vi "MLP Classifier.vi"(8 "error in":errorcluster) -> (0 "error out":errorcluster)   [LabVIEW 2020]
uses:
  <vilib>/Math Plots/3D Math Plots/3D Scatter/3D Scatter XCtrl/3D Scatter.xctl
  Controls/State_MLPClassifier.ctl
  Controls/Local_MLPClassifier.ctl
  Model/Supervised/MultiLayerPerceptron/MLPClassifier/MLPClassifier.lvclass
  C:/Users/cipop/TDF Dropbox/2_Technologies de France/1 - Services et Etudes/PLAIY/2 - DEV/PLAIYLAB/code/Model/Model.lvclass
  C:/Users/cipop/TDF Dropbox/2_Technologies de France/1 - Services et Etudes/PLAIY/2 - DEV/PLAIYLAB/code/Model/Supervised/MultiLayerPerceptron/MultiLayerPerceptron.lvclass
  <vilib>/Math Plots/3D Math Plots/3D Plot/3D Plot Datatype/3D Plot Datatype.lvclass
  PLAIYDISPLAY/Display/Classification/2D/Trained/Controls/2DParameters.ctl
  PLAIYDISPLAY/Display/_Controls/Datas.ctl
  PLAIYDISPLAY/Display/_Controls/PointPropertyMultipleLabel.ctl
  PLAIYDISPLAY/Display/_Controls/Style.ctl
  PLAIYDISPLAY/Display/Classification/3D/_Controls/3DParameters.ctl
  PLAIYDISPLAY/Display/Classification/2D/Predicted/Controls/PredictedParameter.ctl
  88ea5a45-d7b9-4f26-bf7b-97830e46f254.vi
  <vilib>/Utility/file.llb/Application Directory.vi
  <vilib>/Platform/system.llb/System Exec.vi
panel:
  in  "Stop":bool
  in  "TabChoice":enum32{"BTN_Train", "BTN_Predict"}(radio)
  out "Tab Control":enum32{"TRAIN", "PREDICT"}(tab)
  in  "Display_Split":enum16{"All", "Train", "Test"}(ring)
  in  "Representation":u32(ring) items=["2D", "3D"]
  out "GraphTab":enum32{"2D", "3D"}(tab)
  in  "2D":cluster{"X":i32, "Y":i32} {"Y" items=["sepal length (cm)", "sepal width (cm)", "petal length (cm)", "petal width (cm)", "Setosa/Versicolore/Virginica"]; "X" items=["sepal length (cm)", "sepal width (cm)", "petal length (cm)", "petal width (cm)", "Setosa/Versicolore/Virginica"]}
  out "Plot":cluster{"X":dbl[], "Y":dbl[]}[](graph)
  out "CursorTrain":cluster{"Y":dbl, "X":dbl}
  out "3D Scatter":refnum<class "3D Plot Datatype.lvclass">[](xcontrol) caption="Nuage 3D"
  in  "3D":cluster{"X":i32, "Y":i32, "Z":i32} {"Z" items=["sepal length (cm)", "sepal width (cm)", "petal length (cm)", "petal width (cm)", "Setosa/Versicolore/Virginica"]; "Y" items=["sepal length (cm)", "sepal width (cm)", "petal length (cm)", "petal width (cm)", "Setosa/Versicolore/Virginica"]; "X" items=["sepal length (cm)", "sepal width (cm)", "petal length (cm)", "petal width (cm)", "Setosa/Versicolore/Virginica"]}
  in  "%SplitTrain":i32(slide)=50 scale=0.0..100.0 scale format="%#_g %"
  in  "BTN_Train":bool
  in  "BTN_Sauvegarder_M":bool
  in  "BTN_Configurations":bool
  out "Good":i32 caption="Good Prediction"
  out "Bad":i32 caption="Bad Prediction"
  out "Score":dbl caption="Model Score"
  in  "BTN_Predict":bool
  in  "BTN_Load_Model":bool
  in  "PredDisplay":u32(ring) items=["Data", "Graph"]
  out "PredictTab":enum32{"Data", "Graph"}(tab)
  out "Data":dbl[][](array[numeric])
  out "Prediction":dbl[][](array[numeric])
  out "Label":string[](array[string])
  out "GraphPred":cluster{"X":dbl[], "Y":dbl[]}[](graph)
  in  "2D Pred":cluster{"X":i32, "Y":i32}={"X"=0, "Y"=1} {"Y" items=["sepal length (cm)", "sepal width (cm)", "petal length (cm)", "petal width (cm)", "Setosa/Versicolore/Virginica"]; "X" items=["sepal length (cm)", "sepal width (cm)", "petal length (cm)", "petal width (cm)", "Setosa/Versicolore/Virginica"]}
  out "CursorPred":cluster{"Y":dbl, "X":dbl}
  # "MLP Classifier Model - Training"
  # "MLP Classifier Model - Predicting"
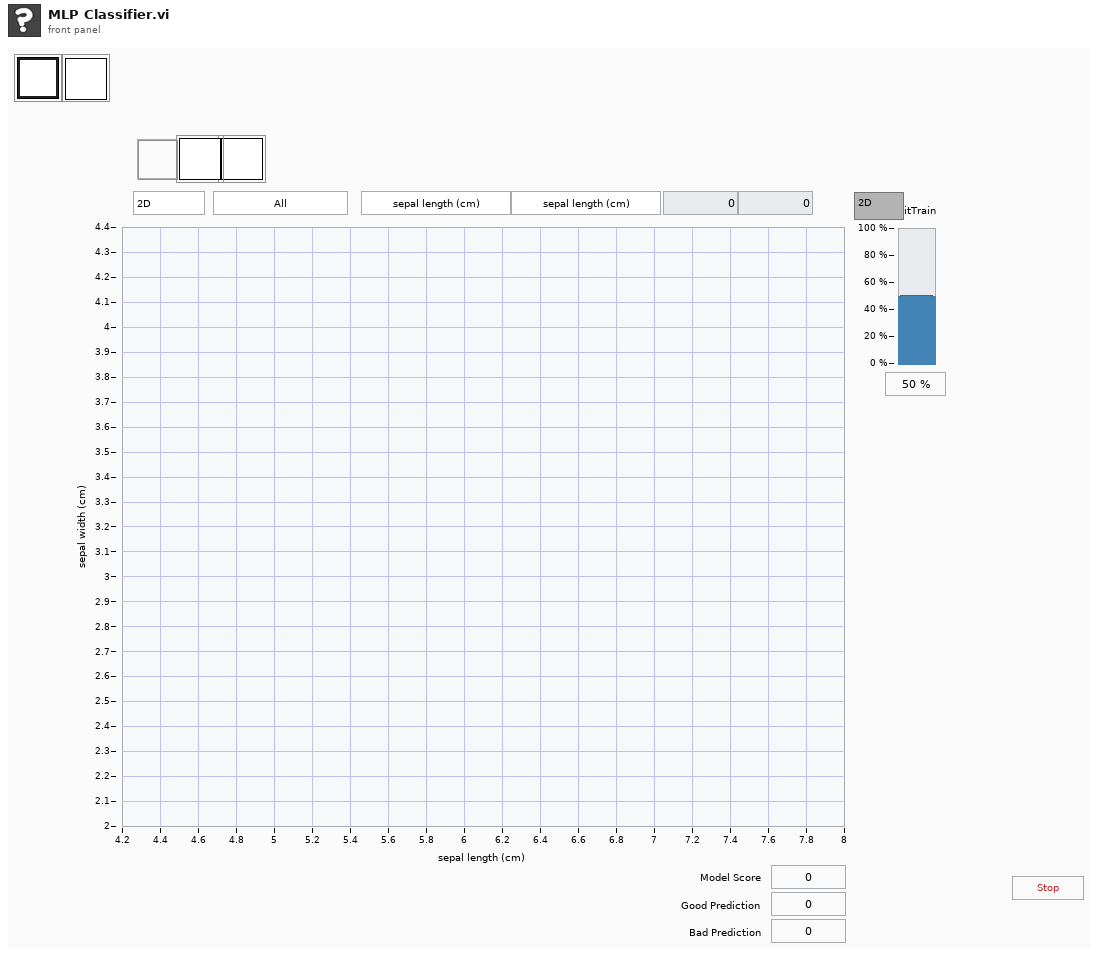
[diagram p1: front panel]
types:
  T1 = typedef "Local_MLPClassifier.ctl" = cluster{"Objet":cluster{"MLPClassifier":refnum<class "MLPClassifier.lvclass">, "3D Plot":refnum<class "3D Plot Datatype.lvclass">[]}, "Référence":cluster{"CursorTrain":refnum<vi>, "GraphPred":refnum<vi>, "GraphTrain":refnum<vi>, "Scale 2D Pred":refnum<vi>, "Scale 3D":refnum<vi>, "Scale 2D":refnum<vi>, "3D Scatter":refnum<vi>, "Data":refnum<vi>, "Prediction":refnum<vi>, "CursorPred":refnum<vi>, "Label":refnum<vi>}, "Variables":cluster{"Mode":enum32{"TRAIN", "PREDICT"}, "Model Name":string, "State":T2, "%SplitTrain":i32, "Representation":u32, "Display_Split":enum16{"All", "Train", "Test"}, "X":dbl[][], "y":dbl[][], "Split":cluster{"X Train":dbl[][], "X Test":dbl[][], "Y Train":dbl[][], "Y Test":dbl[][]}, "FitPredict":dbl[][], "Predict":dbl[][], "ScaleName":string[], "Train ? ":bool}}
  T2 = typedef "State_MLPClassifier.ctl" = enum16{"1 - Idle", "2 - Initialize", "3 - InitializeState", "4 - LoadData", "5 - ScaleName", "6 - SplitTrain", "7 - DisplayDataTrain", "8 - RefreshScale", "9 - Fit", "10 - Predict", "11 - SetParameters", "12 - SaveModel", "13 - LoadModel", "14 - DisplayDataPredict", "Error", "Exit"}
  T3 = typedef "2DParameters.ctl" = cluster{"Plot":refnum<vi>, "Data":T4, "Display":cluster{"Choice":enum16{"All", "Train", "Test"}, "Indexe":cluster{"X":i32, "Y":i32}}, "Property":T5}
  T4 = typedef "Datas.ctl" = cluster{"Split":cluster{"X Train":dbl[][], "X Test":dbl[][], "Y Train":dbl[][], "Y Test":dbl[][]}, "Predict":dbl[][]}
  T5 = typedef "PointPropertyMultipleLabel.ctl" = cluster{"Train Style":T6, "Test OK Style":T6, "Label Color":u32[], "Test NO OK":cluster{"Style":T6, "Color":u32}}
  T6 = typedef "Style.ctl" = enum16{"Empty circle", "Full circle", "Empty square", "Full square", "Cross"}
  T7 = typedef "3DParameters.ctl" = cluster{"3D Plot":refnum<class "3D Plot Datatype.lvclass">[], "3D Scatter":refnum<vi>, "Data":T4, "Display":cluster{"Choice":enum16{"All", "Train", "Test"}, "Indexe":cluster{"X":i32, "Y":i32, "Z":i32}}, "Point Property":T5, "3D Plot Datatype.lvclass":refnum<class "3D Plot Datatype.lvclass">}
  T8 = typedef "PredictedParameter.ctl" = cluster{"Plot":refnum<vi>, "Data":cluster{"X":dbl[][], "Predict":dbl[][]}, "Indexe":cluster{"X":i32, "Y":i32}, "Point Property":cluster{"Style":T6, "Label Color":u32[]}}
  T9 = cluster{"X Train":dbl[][], "X Test":dbl[][], "Y Train":dbl[][], "Y Test":dbl[][]}
  T10 = typedef "mlp_classifier_params.ctl" = cluster{"hidden_layer_sizes":dbl[], "activation":string, "solver":string, "alpha":dbl, "batch_size":cluster{"batch_size_type":string, "batch_size_int":dbl}, "learning_rate":string, "learning_rate_init":dbl, "power_t":dbl, "max_iter":dbl, "shuffle":bool, "random_state":dbl, "tol":dbl, "verbose":bool, "warm_start":bool, "momentum":dbl, "nesterovs_momentum":bool, "early_stopping":bool, "validation_fraction":dbl, "beta_1":dbl, "beta_2":dbl, "epsilon":dbl, "n_iter_no_change":dbl, "max_fun":dbl}
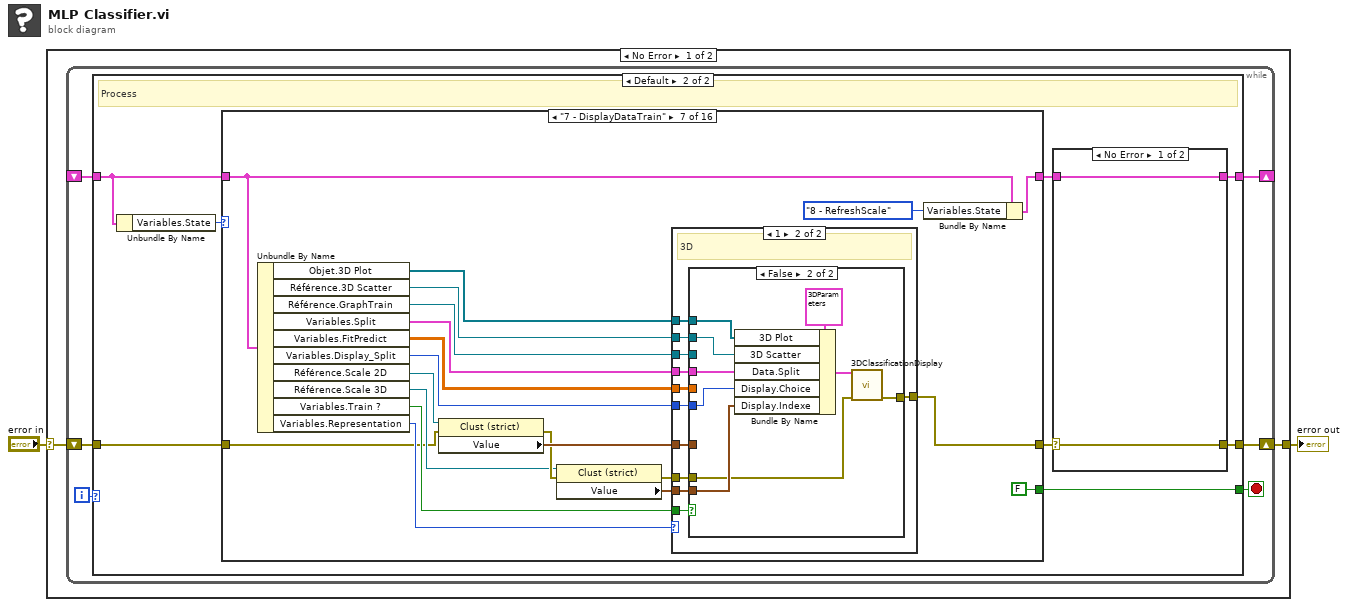
[diagram p0: block diagram]
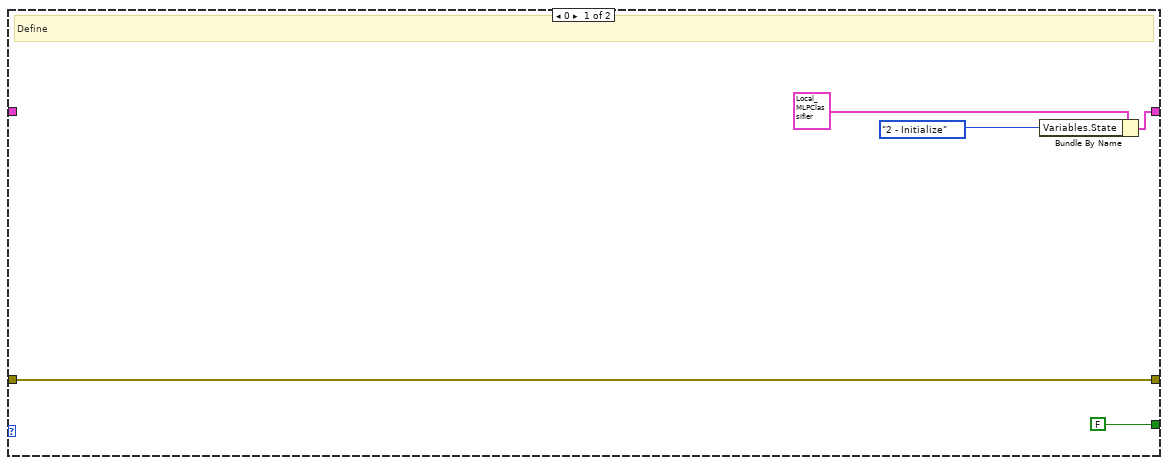
[diagram p2: hidden frame]
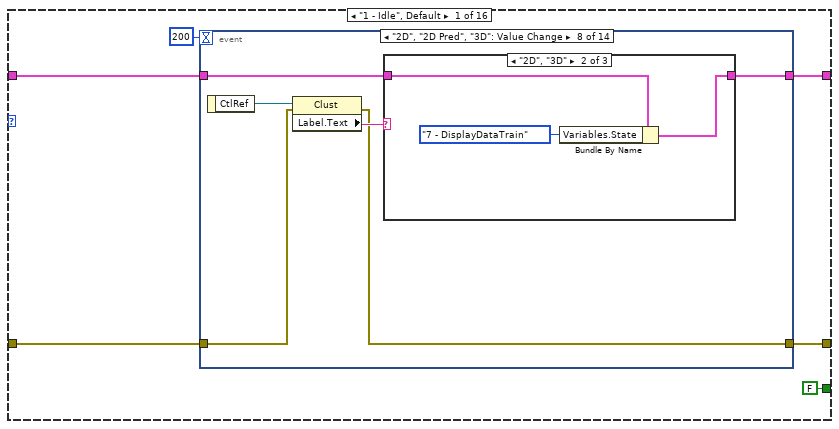
[diagram p3: hidden frame]
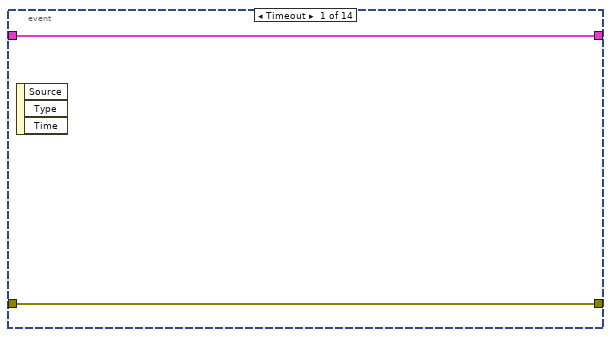
[diagram p4: hidden frame]
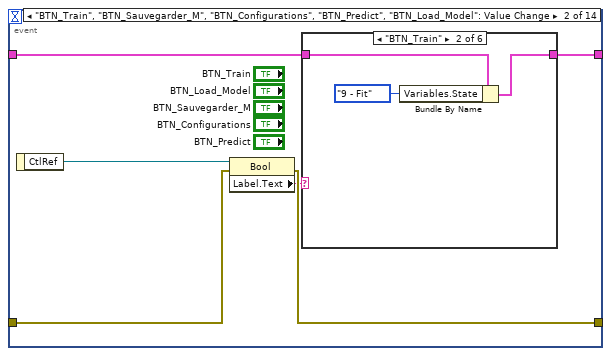
[diagram p5: hidden frame]
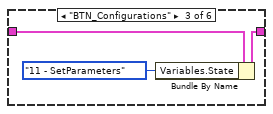
[diagram p7: hidden frame]
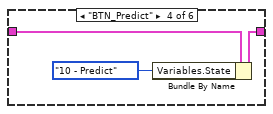
[diagram p8: hidden frame]
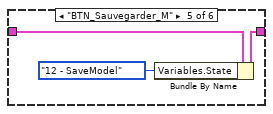
[diagram p9: hidden frame]
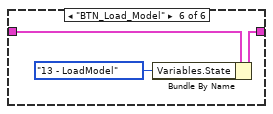
[diagram p10: hidden frame]
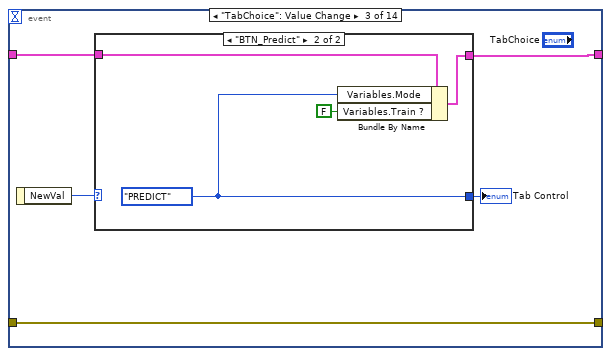
[diagram p11: hidden frame]
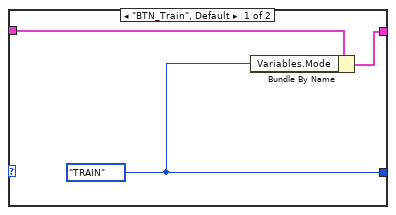
[diagram p12: hidden frame]
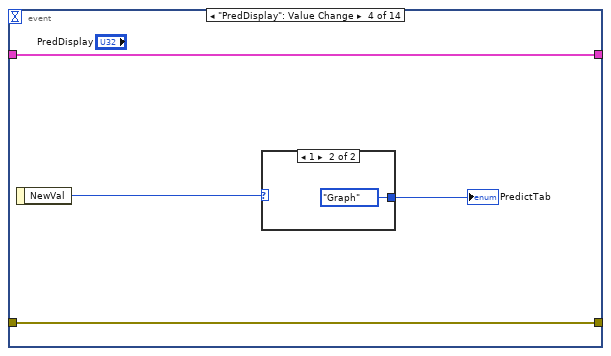
[diagram p13: hidden frame]
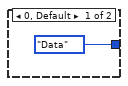
[diagram p14: hidden frame]
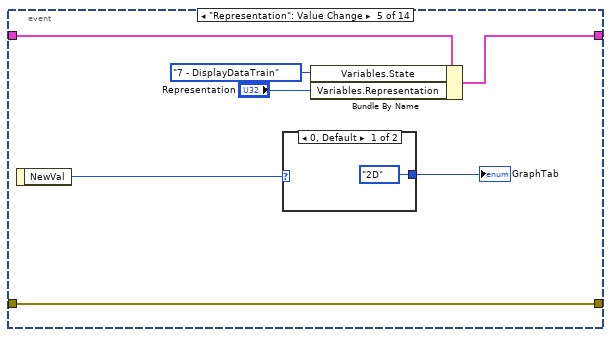
[diagram p15: hidden frame]
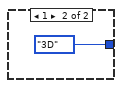
[diagram p16: hidden frame]
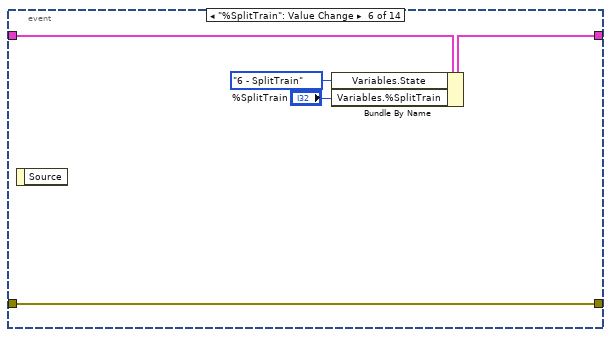
[diagram p17: hidden frame]
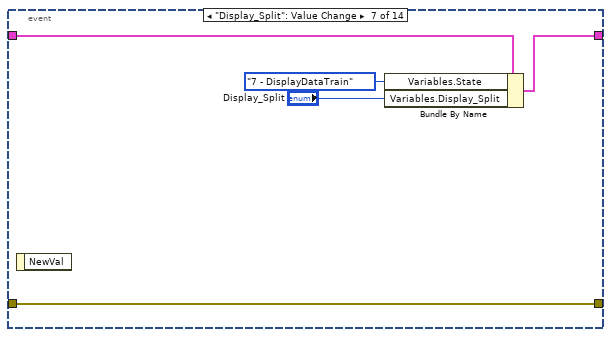
[diagram p18: hidden frame]
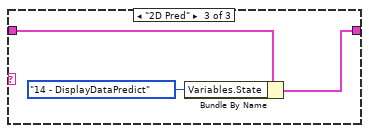
[diagram p20: hidden frame]
diagram:
  n1 = case shown="No Error" "error in" {
    selector: "error in" -> [w4 w673]
    tunnel: [w3 w673] -> w1
    frame No Error {
      n2 = while {
        shift-right: [w9] -> w3
        shift-left: w4 -> [w10]
        shift-right: [w5] -> _
        shift-left: _ -> [w6]
        i -> [w7]
        stop <- w8 stop-if-true
        n3 = case shown="Default" w7 {
          tunnel: w10 -> [w15 w23]
          tunnel: w6 -> [_ w22]
          tunnel: [w15 w20] -> w9
          tunnel: [FALSE w19] -> w8
          tunnel: [w11 w16] -> w5
          frame 0 {
            # "Define"
            n4 = Bundle By Name(cluster=T1 {"Objet"={"MLPClassifier"=refnum, "3D Plot"=[]}, "Référence"={"CursorTrain"=refnum, "GraphPred"=refnum, "GraphTrain"=refnum, "Scale 2D Pred"=refnum, "Scale 3D"=refnum, "Scale 2D"=refnum, "3D Scatter"=refnum, "Data"=refnum, "Prediction"=refnum, "CursorPred"=refnum, "Label"=refnum}, "Variables"={"Mode"=enum."TRAIN", "Model Name"="", "State"=enum."3 - InitializeState", "%SplitTrain"=5, "Representation"=0, "Display_Split"=enum."All", "X"=[], "y"=[], "Split"={"X Train"=[], "X Test"=[], "Y Train"=[], "Y Test"=[]}, "FitPredict"=[], "Predict"=[], "ScaleName"=[], "Train ? "=FALSE}} ("Local"), "Variables.State"=State_MLPClassifier."2 - Initialize" ("Enum")) -> (w11:T1)
          }
          frame Default {
            # "Process"
            n5 = Unbundle By Name(w22) -> ("Variables.State"=w18:T2)
            n6 = case shown="\"7 - DisplayDataTrain\"" w18 {
              tunnel: w23 -> [w29 w169 w191 w202 w238 w347 w353 w436 w494 w508 w551 w571 w602 w627 w643 w664]
              tunnel: w22 -> [w27 w170 w190 w205 w235 w350 w354 w433 w496 w510 w552 w559 w593 w639 w644 w662]
              tunnel: [w28 w165 w183 w201 w236 w346 w371 w435 w498 w512 w550 w570 w603 w628 w646 w663] -> w21
              tunnel: [FALSE FALSE FALSE FALSE FALSE FALSE FALSE FALSE FALSE FALSE FALSE FALSE FALSE FALSE FALSE TRUE] -> w19
              tunnel: [w24 w151 w177 w200 w234 w344 w367 w432 w493 w511 w548 w566 w592 w638 w642 w662] -> w17
              frame "1 - Idle", Default {
                n7 = event shown="[7] \"2D\", \"2D Pred\", \"3D\": Value Change" {
                  selector: _ -> [_ _ _ _ _ _ _ _ _ _ _ _ _ _]
                  dyn-events: _ -> [_ _ _ _ _ _ _ _ _ _ _ _ _ _]
                  timeout: 200 -> [_ _ _ _ _ _ _ _ _ _ _ _ _ _]
                  tunnel: w29 -> [w31 w32 w58 w68 w78 w82 w87 w92 w109 w118 w120 w125 w130 w150]
                  tunnel: [w31 w34 w58 w68 w78 w82 w87 w91 w105 w112 w121 w126 w132 w150] -> w28
                  tunnel: w27 -> [w30 w37 w54 w69 w75 w85 w90 w96 w104 w111 w123 w128 w131 w149]
                  tunnel: [w30 w36 w55 w69 w74 w84 w89 w95 w104 w111 w123 w128 w131 w148] -> w24
                  event Timeout {
                    n8 = event-data() -> ()  [unwired: 1 in, 3 out]
                  }
                  event "BTN_Train", "BTN_Sauvegarder_M", "BTN_Configurations", "BTN_Predict", "BTN_Load_Model": Value Change {
                    n9 = event-data() -> ("CtlRef"=w35:refnum<vi>)  [unwired: 1 in]
                    n10 = property class="Bool"(reference=w35, error in=w32) -> (error out=w34:errorcluster, "Label.Text"=w33:string)  [unwired: 1 out]
                    n11 = case shown="\"BTN_Train\"" w33 {
                      tunnel: w37 -> [w38 w41 w44 w47 w50 w53]
                      tunnel: [w38 w40 w43 w46 w49 w52] -> w36
                      frame Default {
                      }
                      frame "BTN_Train" {
                        n12 = Bundle By Name(cluster=w41, "Variables.State"=State_MLPClassifier."9 - Fit") -> (w40:T1)
                      }
                      frame "BTN_Configurations" {
                        n13 = Bundle By Name(cluster=w44, "Variables.State"=State_MLPClassifier."11 - SetParameters") -> (w43:T1)
                      }
                      frame "BTN_Predict" {
                        n14 = Bundle By Name(cluster=w47, "Variables.State"=State_MLPClassifier."10 - Predict") -> (w46:T1)
                      }
                      frame "BTN_Sauvegarder_M" {
                        n15 = Bundle By Name(cluster=w50, "Variables.State"=State_MLPClassifier."12 - SaveModel") -> (w49:T1)
                      }
                      frame "BTN_Load_Model" {
                        n16 = Bundle By Name(cluster=w53, "Variables.State"=State_MLPClassifier."13 - LoadModel") -> (w52:T1)
                      }
                    }
                  }
                  event "TabChoice": Value Change {
                    n17 = event-data() -> ("NewVal"=w57:enum32{"BTN_Train", "BTN_Predict"})  [unwired: 1 in]
                    n18 = case shown="\"BTN_Predict\"" w57 {
                      tunnel: [w59 w65] -> w56
                      tunnel: [w60 w64] -> w55
                      tunnel: w54 -> [w61 w63]
                      frame "BTN_Train", Default {
                        w59 = enum32{"TRAIN", "PREDICT"}."TRAIN" ("Tab Control")
                        n19 = Bundle By Name(cluster=w61, "Variables.Mode"=w59) -> (w60:T1)
                      }
                      frame "BTN_Predict" {
                        w65 = enum32{"TRAIN", "PREDICT"}."PREDICT" ("Tab Control")
                        n20 = Bundle By Name(cluster=w63, "Variables.Mode"=w65, "Variables.Train ?"=FALSE) -> (w64:T1)
                      }
                    }
                    "Tab Control" <- w56
                  }
                  event "PredDisplay": Value Change {
                    n21 = event-data() -> ("NewVal"=w67:u32)  [unwired: 1 in]
                    n22 = case shown="1" w67 {
                      tunnel: [enum32{"Data", "Graph"}."Data" ("PredictTab") enum32{"Data", "Graph"}."Graph" ("PredictTab")] -> w66
                      frame 0, Default {
                      }
                      frame 1 {
                      }
                    }
                    "PredictTab" <- w66
                  }
                  event "Representation": Value Change {
                    n23 = event-data() -> ("NewVal"=w77:u32)  [unwired: 1 in]
                    n24 = case shown="0, Default" w77 {
                      tunnel: [enum32{"2D", "3D"}."2D" ("GraphTab") enum32{"2D", "3D"}."3D" ("GraphTab")] -> w76
                      frame 0, Default {
                      }
                      frame 1 {
                      }
                    }
                    "GraphTab" <- w76
                    n25 = Bundle By Name(cluster=w75, "Variables.State"=State_MLPClassifier."7 - DisplayDataTrain", "Variables.Representation"="Representation") -> (w74:T1)
                  }
                  event "%SplitTrain": Value Change {
                    n26 = event-data() -> ()  [unwired: 1 in, 1 out]
                    n27 = Bundle By Name(cluster=w85, "Variables.State"=State_MLPClassifier."6 - SplitTrain", "Variables.%SplitTrain"="%SplitTrain") -> (w84:T1)
                  }
                  event "Display_Split": Value Change {
                    n28 = event-data() -> ()  [unwired: 1 in, 1 out]
                    n29 = Bundle By Name(cluster=w90, "Variables.State"=State_MLPClassifier."7 - DisplayDataTrain", "Variables.Display_Split"="Display_Split") -> (w89:T1)
                  }
                  event "2D", "2D Pred", "3D": Value Change {
                    n30 = event-data() -> ("CtlRef"=w94:refnum<vi>)  [unwired: 1 in]
                    n31 = property class="Clust"(reference=w94, error in=w92) -> (error out=w91:errorcluster, "Label.Text"=w93:string)  [unwired: 1 out]
                    n32 = case shown="\"2D\", \"3D\"" w93 {
                      tunnel: w96 -> [w97 w100 w103]
                      tunnel: [w97 w99 w102] -> w95
                      frame Default {
                      }
                      frame "2D", "3D" {
                        n33 = Bundle By Name(cluster=w100, "Variables.State"=State_MLPClassifier."7 - DisplayDataTrain") -> (w99:T1)
                      }
                      frame "2D Pred" {
                        n34 = Bundle By Name(cluster=w103, "Variables.State"=State_MLPClassifier."14 - DisplayDataPredict") -> (w102:T1)
                      }
                    }
                  }
                  event "Prediction": Mouse Up; "Prediction": Mouse Wheel; "Prediction": Mouse Leave {
                    n35 = event-data() -> ()  [unwired: 1 in, 1 out]
                    n36 = Unbundle By Name(w104) -> ("Référence.Prediction"=w110:refnum<vi>, "Référence.Data"=w108:refnum<vi>)
                    n37 = property class="Arr (strict)"(reference=w110, error in=w109) -> (error out=w106:errorcluster, "Index Values"=w107:u32[])  [unwired: 1 out]
                    n38 = property class="Arr (strict)"(reference=w108, error in=w106, "Index Values"=w107) -> (error out=w105:errorcluster)  [unwired: 1 out]
                  }
                  event "Data": Mouse Up; "Data": Mouse Wheel; "Data": Mouse Leave {
                    n39 = event-data() -> ()  [unwired: 1 in, 1 out]
                    n40 = Unbundle By Name(w111) -> ("Référence.Data"=w119:refnum<vi>, "Référence.Label"=w117:refnum<vi>)
                    n41 = property class="Arr (strict)"(reference=w119, error in=w118) -> (error out=w113:errorcluster, "Index Values"=w114:u32[])  [unwired: 1 out]
                    n42 = Rotate 1D Array(1:w114, 2:1 ("n")) -> (0:w115:u32[])
                    n43 = property class="Arr (strict)"(reference=w117, error in=w113, "Index Values"=w115) -> (error out=w112:errorcluster)  [unwired: 1 out]
                  }
                  event "GraphPred", "Plot": Mouse Enter {
                    n44 = event-data() -> ("CtlRef"=w124:refnum<vi>)  [unwired: 1 in]
                    n45 = property class="XYGraph (strict)"(reference=w124, error in=w120, "Cursor.Visible"=TRUE) -> (error out=w121:errorcluster)  [unwired: 1 out]
                  }
                  event "GraphPred", "Plot": Mouse Leave {
                    n46 = event-data() -> ("CtlRef"=w129:refnum<vi>)  [unwired: 1 in]
                    n47 = property class="XYGraph (strict)"(reference=w129, error in=w125, "Cursor.Visible"=FALSE) -> (error out=w126:errorcluster)  [unwired: 1 out]
                  }
                  event "GraphPred", "Plot": Cursor Move {
                    n48 = event-data() -> ("CursLoc"=w134:cluster{"X":dbl, "Y":dbl}, "CtlRef"=w138:refnum<vi>)  [unwired: 1 in]
                    n49 = property class="XYGraph (strict)"(reference=w138, error in=w130) -> (error out=w133:errorcluster, "Label.Text"=w137:string)  [unwired: 1 out]
                    n50 = Unbundle By Name(w131) -> ("Référence.CursorTrain"=w136:refnum<vi>, "Référence.CursorPred"=w135:refnum<vi>)
                    n51 = case shown="\"GraphTrain\", Default" w137 {
                      tunnel: w134 -> [w141 w146]
                      tunnel: w136 -> [_ w143]
                      tunnel: w135 -> [w142 _]
                      tunnel: w133 -> [w140 w145]
                      tunnel: [w139 w144] -> w132
                      frame "GraphPred" {
                        n52 = property class="Clust (strict)"(reference=w142, error in=w140, "Value"=w141) -> (error out=w139:errorcluster)  [unwired: 1 out]
                      }
                      frame "GraphTrain", Default {
                        n53 = property class="Clust (strict)"(reference=w143, error in=w145, "Value"=w146) -> (error out=w144:errorcluster)  [unwired: 1 out]
                      }
                    }
                  }
                  event "Stop": Value Change {
                    n54 = event-data() -> ()  [unwired: 1 in, 6 out]
                    n55 = Bundle By Name(cluster=w149, "Variables.State"=State_MLPClassifier."Exit" ("State")) -> (w148:T1)
                  }
                }
              }
              frame "2 - Initialize" {
                n56 = call "MLPClassifier.vi"("error in"=w169) -> ("error out"=w166:errorcluster, "out"=w168:refnum<class "MLPClassifier.lvclass">)  [unwired: 9 in]
                n57 = call-dynamic "init.vi"("error in (no error)"=w166, "Model en entrée"=w168) -> ("error out"=w165:errorcluster, "Model en sortie"=w167:refnum<class "MLPClassifier.lvclass">)  [unwired: 8 in]
                n58 = control-ref of="3D Scatter"() -> (w156:refnum<vi>)
                n59 = control-ref of="GraphPred"() -> (w161:refnum<vi>)
                n60 = control-ref of="Plot"() -> (w162:refnum<vi>)
                n61 = control-ref of="CursorPred"() -> (w153:refnum<vi>)
                n62 = control-ref of="Scale 2D Pred"() -> (w158:refnum<vi>)
                n63 = control-ref of="Scale 3D"() -> (w159:refnum<vi>)
                n64 = control-ref of="Scale 2D"() -> (w160:refnum<vi>)
                n65 = control-ref of="CursorTrain"() -> (w163:refnum<vi>)
                n66 = control-ref of="Label"() -> (w152:refnum<vi>)
                n67 = control-ref of="Data"() -> (w154:refnum<vi>)
                n68 = control-ref of="Prediction"() -> (w155:refnum<vi>)
                n69 = Bundle By Name(cluster=w170, "Référence.Label"=w152, "Référence.CursorPred"=w153, "Référence.Data"=w154, "Référence.Prediction"=w155, "Référence.3D Scatter"=w156, "Référence.Scale 2D Pred"=w158, "Référence.Scale 3D"=w159, "Référence.Scale 2D"=w160, "Référence.GraphPred"=w161, "Référence.GraphTrain"=w162, "Référence.CursorTrain"=w163, "Objet.3D Plot"=refnum<class "3D Plot Datatype.lvclass">[] [] ("3D Plot lvclass Array out"), "Variables.State"=State_MLPClassifier."3 - InitializeState", "Objet.MLPClassifier"=w167) -> (w151:T1)
              }
              frame "3 - InitializeState" {
                n70 = Unbundle By Name(w190) -> ("Objet.MLPClassifier"=w176:refnum<class "MLPClassifier.lvclass">, "Référence.Data"=w189:refnum<vi>, "Référence.Prediction"=w188:refnum<vi>, "Référence.Label"=w186:refnum<vi>)
                n71 = invoke class="VI" method="Default Vals.Reinit All"(error in=w191) -> (error out=w175:errorcluster)  [unwired: 2 in, 2 out]
                n72 = property class="MLPClassifier.lvclass"(reference=w176, error in=w175) -> (reference out=w172:refnum<class "MLPClassifier.lvclass">, error out=w173:errorcluster, "accessors:R/W name"=w174:string)
                n73 = property class="Arr (strict)"(reference=w189, error in=w175, "Index Values"=u32[] [0]) -> (error out=w182:errorcluster)  [unwired: 1 out]
                n74 = property class="Arr (strict)"(reference=w188, error in=w175, "Index Values"=u32[] [0]) -> (error out=w181:errorcluster)  [unwired: 1 out]
                n75 = property class="Arr (strict)"(reference=w186, error in=w175, "Index Values"=u32[] [0]) -> (error out=w180:errorcluster)  [unwired: 1 out]
                n76 = Bundle By Name(cluster=w190, "Objet.MLPClassifier"=w172, "Variables.State"=State_MLPClassifier."4 - LoadData" ("State"), "Variables.%SplitTrain"=50, "Variables.Model Name"=w174, "Variables.Mode"=enum32{"TRAIN", "PREDICT"}."TRAIN") -> (w177:T1)
                n77 = Merge Errors(w173, w182, w181, w180) -> (w183:errorcluster)
              }
              frame "4 - LoadData" {
                # "Transform strings into doubles"
                # "Separate X from y"
                n78 = call "Load_Iris.vi"("error in"=w202) -> ("error out"=w203:errorcluster, "Tableau"=w208:string[][])  [unwired: 9 in]
                n79 = Index Array(array=w208, index (row)=0) -> (element=w204:string[])  [unwired: 1 in]
                n80 = Array Subset(array=w208, index (row)=1 ("index"), length (col)=4 ("length")) -> (w221:string[][])  [unwired: 2 in]
                n81 = Array Subset(array=w208, index (row)=1 ("index"), index (col)=4 ("index")) -> (w212:string[][])  [unwired: 2 in]
                n82 = for {
                  tunnel: w204 -> [w232] mode=indexing
                  tunnel: [w230] -> w196 mode=indexing
                  shift-right: [w227] -> w201
                  shift-left: w203 -> [w228]
                  n83 = Search and Replace String(replace all?=TRUE ("replace all? (F)"), input string=w232, search string="'", error in=w228) -> (result string=w230:string, error out=w227:errorcluster)  [unwired: 4 in, 2 out]
                }
                n84 = Array To Spreadsheet String(delimiter (Tab)=";", array=w212, 3:"%s" ("format string")) -> (spreadsheet string=w213:string)
                n85 = Array To Spreadsheet String(delimiter (Tab)=";", array=w221, 3:"%s" ("format string")) -> (spreadsheet string=w217:string)
                n86 = Spreadsheet String To Array(delimiter (Tab)=";", format string="%.;%#g", spreadsheet string=w213) -> (array=w209:dbl[][])  [unwired: 1 in]
                n87 = Spreadsheet String To Array(delimiter (Tab)=";", format string="%.;%#g", spreadsheet string=w217) -> (array=w199:dbl[][])  [unwired: 1 in]
                "Data" <- w199
                n88 = Array Size(array=w196) -> (size(s)=w198:i32)
                n89 = Subtract(x=w198, y=1) -> (x-y=w195:i32)
                n90 = Delete From Array(array=w196, index=w195) -> (array with subset deleted=→"Label":string[])  [unwired: 1 in, 1 out]
                n91 = Bundle By Name(cluster=w205, "Variables.ScaleName"=w196, "Variables.State"=State_MLPClassifier."5 - ScaleName", "Variables.X"=w199, "Variables.y"=w209) -> (w200:T1)
              }
              frame "5 - ScaleName" {
                n92 = Unbundle By Name(w235) -> ("Variables.Mode"=w237:enum32{"TRAIN", "PREDICT"}, "Variables.ScaleName"=w239:string[], "Référence.Scale 2D Pred"=w242:refnum<vi>, "Référence.Scale 3D"=w241:refnum<vi>, "Référence.Scale 2D"=w240:refnum<vi>)
                n93 = case shown="\"PREDICT\"" w237 {
                  tunnel: w242 -> [w253 _]
                  tunnel: w241 -> [_ w288]
                  tunnel: w240 -> [_ w285]
                  tunnel: w239 -> [w246 w283]
                  tunnel: w238 -> [w250 w284]
                  tunnel: [w249 w280] -> w236
                  tunnel: w235 -> [w248 w279]
                  tunnel: [w247 w277] -> w234
                  tunnel: refnum<vi> refnum ("X 2") -> [w244 w276]
                  frame "PREDICT" {
                    n94 = property class="Clust (strict)"(reference=w253, error in=w250) -> (error out=w251:errorcluster, "Controls[]"=w252:refnum<vi>[])  [unwired: 1 out]
                    n95 = for {
                      tunnel: w252 -> [w259] mode=indexing
                      tunnel: w244 -> [w258]
                      shift-right: [w256] -> w249
                      shift-left: w251 -> [w257]
                      tunnel: w246 -> [w255]
                      i -> [w254]
                      n96 = case shown="1" w254 {
                        tunnel: w259 -> [w267 w275]
                        tunnel: w258 -> [w266 w274]
                        tunnel: w257 -> [w264 w272]
                        tunnel: [w262 w270] -> w256
                        tunnel: w255 -> [w261 w269]
                        frame 0, Default {
                          n97 = To More Specific Class(target class=w266, reference=w267, error in=w264) -> (specific class reference=w265:refnum<vi>, error out=w263:errorcluster)
                          n98 = property class="Ring (strict)"(reference=w265, error in=w263, "Strings []"=w261, "Value"=0) -> (error out=w262:errorcluster)  [unwired: 1 out]
                        }
                        frame 1 {
                          n99 = To More Specific Class(target class=w274, reference=w275, error in=w272) -> (specific class reference=w273:refnum<vi>, error out=w271:errorcluster)
                          n100 = property class="Ring (strict)"(reference=w273, error in=w271, "Strings []"=w269, "Value"=1) -> (error out=w270:errorcluster)  [unwired: 1 out]
                        }
                      }
                    }
                    n101 = Bundle By Name(cluster=w248, "Variables.State"=State_MLPClassifier."14 - DisplayDataPredict") -> (w247:T1)
                  }
                  frame "TRAIN", Default {
                    n102 = property class="Clust (strict)"(reference=w288, error in=w284) -> (error out=w290:errorcluster, "Controls[]"=w289:refnum<vi>[])  [unwired: 1 out]
                    n103 = property class="Clust (strict)"(reference=w285, error in=w284) -> (error out=w286:errorcluster, "Controls[]"=w287:refnum<vi>[])  [unwired: 1 out]
                    n104 = for {
                      tunnel: w289 -> [w318] mode=indexing
                      shift-right: [w316] -> w281
                      shift-left: w290 -> [w317]
                      tunnel: w283 -> [w315]
                      tunnel: w276 -> [w313]
                      i -> [w314]
                      n105 = case shown="1" w314 {
                        tunnel: w318 -> [w326 w334 w342]
                        tunnel: w313 -> [w325 w333 w341]
                        tunnel: w317 -> [w323 w331 w339]
                        tunnel: [w321 w329 w337] -> w316
                        tunnel: w315 -> [w320 w328 w336]
                        frame 0, Default {
                          n106 = To More Specific Class(target class=w325, reference=w326, error in=w323) -> (specific class reference=w324:refnum<vi>, error out=w322:errorcluster)
                          n107 = property class="Ring (strict)"(reference=w324, error in=w322, "Strings []"=w320, "Value"=0) -> (error out=w321:errorcluster)  [unwired: 1 out]
                        }
                        frame 1 {
                          n108 = To More Specific Class(target class=w333, reference=w334, error in=w331) -> (specific class reference=w332:refnum<vi>, error out=w330:errorcluster)
                          n109 = property class="Ring (strict)"(reference=w332, error in=w330, "Strings []"=w328, "Value"=1) -> (error out=w329:errorcluster)  [unwired: 1 out]
                        }
                        frame 2 {
                          n110 = To More Specific Class(target class=w341, reference=w342, error in=w339) -> (specific class reference=w340:refnum<vi>, error out=w338:errorcluster)
                          n111 = property class="Ring (strict)"(reference=w340, error in=w338, "Strings []"=w336, "Value"=2) -> (error out=w337:errorcluster)  [unwired: 1 out]
                        }
                      }
                    }
                    n112 = for {
                      tunnel: w287 -> [w296] mode=indexing
                      shift-right: [w294] -> w282
                      shift-left: w286 -> [w295]
                      tunnel: w283 -> [w293]
                      tunnel: w276 -> [w291]
                      i -> [w292]
                      n113 = case shown="1" w292 {
                        tunnel: w296 -> [w304 w312]
                        tunnel: w291 -> [w303 w311]
                        tunnel: w295 -> [w301 w309]
                        tunnel: [w299 w307] -> w294
                        tunnel: w293 -> [w298 w306]
                        frame 0, Default {
                          n114 = To More Specific Class(target class=w303, reference=w304, error in=w301) -> (specific class reference=w302:refnum<vi>, error out=w300:errorcluster)
                          n115 = property class="Ring (strict)"(reference=w302, error in=w300, "Strings []"=w298, "Value"=0) -> (error out=w299:errorcluster)  [unwired: 1 out]
                        }
                        frame 1 {
                          n116 = To More Specific Class(target class=w311, reference=w312, error in=w309) -> (specific class reference=w310:refnum<vi>, error out=w308:errorcluster)
                          n117 = property class="Ring (strict)"(reference=w310, error in=w308, "Strings []"=w306, "Value"=1) -> (error out=w307:errorcluster)  [unwired: 1 out]
                        }
                      }
                    }
                    n118 = Bundle By Name(cluster=w279, "Variables.State"=State_MLPClassifier."6 - SplitTrain") -> (w277:T1)
                    n119 = Merge Errors(w281, w282) -> (w280:errorcluster)
                  }
                }
              }
              frame "6 - SplitTrain" {
                n120 = Unbundle By Name(w350) -> ("Variables.%SplitTrain"=w348:i32, "Variables.X"=w352:dbl[][], "Variables.y"=w351:dbl[][])
                n121 = call "SplitDataSetXY.vi"("%SplitTrain"=w348, "error in (no error)"=w347, "Y"=w351, "X"=w352) -> ("error out"=w346:errorcluster, "Split"=w345:T9)  [unwired: 6 in]
                n122 = Bundle By Name(cluster=w350, "Variables.State"=State_MLPClassifier."7 - DisplayDataTrain", "Variables.Split"=w345) -> (w344:T1)
              }
              frame "7 - DisplayDataTrain" {
                n123 = Unbundle By Name(w354) -> ("Objet.3D Plot"=w362:refnum<class "3D Plot Datatype.lvclass">[], "Référence.3D Scatter"=w366:refnum<vi>, "Référence.GraphTrain"=w365:refnum<vi>, "Variables.Split"=w364:T9, "Variables.FitPredict"=w363:dbl[][], "Variables.Display_Split"=w361:enum16{"All", "Train", "Test"}, "Référence.Scale 2D"=w360:refnum<vi>, "Référence.Scale 3D"=w355:refnum<vi>, "Variables.Train ?"=w370:bool, "Variables.Representation"=w368:u32)
                n124 = property class="Clust (strict)"(reference=w360, error in=w353) -> (error out=w358:errorcluster, "Value"=w359:cluster{"X":i32, "Y":i32})  [unwired: 1 out]
                n125 = property class="Clust (strict)"(reference=w355, error in=w358) -> (error out=w357:errorcluster, "Value"=w356:cluster{"X":i32, "Y":i32, "Z":i32})  [unwired: 1 out]
                n126 = case shown="1" w368 {
                  tunnel: [w383 w405] -> w371
                  tunnel: w370 -> [w382 w411]
                  tunnel: w366 -> [w381 w407]
                  tunnel: w365 -> [w380 w408]
                  tunnel: w364 -> [w379 w409]
                  tunnel: w363 -> [w378 w410]
                  tunnel: w362 -> [w376 w406]
                  tunnel: w361 -> [w377 w404]
                  tunnel: w359 -> [w374 w403]
                  tunnel: w357 -> [w375 w402]
                  tunnel: w356 -> [w373 w401]
                  frame 0, Default {
                    # "2D"
                    n127 = case shown="True" w382 {
                      tunnel: [w387 w392] -> w383
                      tunnel: w381 -> [_ _]
                      tunnel: w380 -> [w391 w400]
                      tunnel: w379 -> [w390 w399]
                      tunnel: w378 -> [_ w398]
                      tunnel: w377 -> [w389 w397]
                      tunnel: w376 -> [_ _]
                      tunnel: w375 -> [w386 w393]
                      tunnel: w374 -> [w388 w396]
                      tunnel: w373 -> [_ _]
                      frame False {
                        n128 = Bundle By Name(cluster=T3 {"Plot"=refnum, "Data"={"Split"={"X Train"=[], "X Test"=[], "Y Train"=[], "Y Test"=[]}, "Predict"=[]}, "Display"={"Choice"=enum."All", "Indexe"={"X"=0, "Y"=1}}, "Property"={"Train Style"=enum."Full circle", "Test OK Style"=enum."Full square", "Label Color"=[8978528, 4367871, 1985280], "Test NO OK"={"Style"=enum."Cross", "Color"=16716800}}} ("Parameters"), "Plot"=w391, "Data.Split"=w390, "Display.Choice"=w389, "Display.Indexe"=w388) -> (w384:T3)
                        n129 = call "2DClassificationDisplay.vi"("error in"=w386, "Parameters"=w384) -> ("error out"=w387:errorcluster)  [unwired: 9 in]
                      }
                      frame True {
                        n130 = Bundle By Name(cluster=T3 {"Plot"=refnum, "Data"={"Split"={"X Train"=[], "X Test"=[], "Y Train"=[], "Y Test"=[]}, "Predict"=[]}, "Display"={"Choice"=enum."All", "Indexe"={"X"=0, "Y"=1}}, "Property"={"Train Style"=enum."Full circle", "Test OK Style"=enum."Full square", "Label Color"=[8978528, 4367871, 1985280], "Test NO OK"={"Style"=enum."Cross", "Color"=16716800}}} ("Parameters"), "Plot"=w400, "Data.Split"=w399, "Data.Predict"=w398, "Display.Choice"=w397, "Display.Indexe"=w396) -> (w394:T3)
                        n131 = call "2DClassificationDisplay.vi"("error in"=w393, "Parameters"=w394) -> ("error out"=w392:errorcluster)  [unwired: 9 in]
                      }
                    }
                  }
                  frame 1 {
                    # "3D"
                    n132 = case shown="False" w411 {
                      tunnel: [w412 w423] -> w405
                      tunnel: w408 -> [_ _]
                      tunnel: w409 -> [w421 w430]
                      tunnel: w410 -> [w420 _]
                      tunnel: w407 -> [w418 w428]
                      tunnel: w406 -> [w419 w429]
                      tunnel: w404 -> [w417 w427]
                      tunnel: w403 -> [_ _]
                      tunnel: w402 -> [w414 w424]
                      tunnel: w401 -> [w416 w426]
                      frame True {
                        n133 = Bundle By Name(cluster=T7 {"3D Plot"=[], "3D Scatter"=refnum, "Data"={"Split"={"X Train"=[], "X Test"=[], "Y Train"=[], "Y Test"=[]}, "Predict"=[]}, "Display"={"Choice"=enum."All", "Indexe"={"X"=0, "Y"=1, "Z"=2}}, "Point Property"={"Train Style"=enum."Full circle", "Test OK Style"=enum."Full square", "Label Color"=[8978528, 4367871, 1985280], "Test NO OK"={"Style"=enum."Cross", "Color"=16716800}}, "3D Plot Datatype.lvclass"=refnum} ("Parameter"), "3D Plot"=w419, "3D Scatter"=w418, "Data.Split"=w421, "Data.Predict"=w420, "Display.Choice"=w417, "Display.Indexe"=w416) -> (w413:T7)
                        n134 = call "3DClassificationDisplay.vi"("error in"=w414, "Parameter"=w413) -> ("error out"=w412:errorcluster)  [unwired: 9 in]
                      }
                      frame False {
                        n135 = Bundle By Name(cluster=T7 {"3D Plot"=[], "3D Scatter"=refnum, "Data"={"Split"={"X Train"=[], "X Test"=[], "Y Train"=[], "Y Test"=[]}, "Predict"=[]}, "Display"={"Choice"=enum."All", "Indexe"={"X"=0, "Y"=1, "Z"=2}}, "Point Property"={"Train Style"=enum."Full circle", "Test OK Style"=enum."Full square", "Label Color"=[8978528, 4367871, 1985280], "Test NO OK"={"Style"=enum."Cross", "Color"=16716800}}, "3D Plot Datatype.lvclass"=refnum} ("Parameter"), "3D Plot"=w429, "3D Scatter"=w428, "Data.Split"=w430, "Display.Choice"=w427, "Display.Indexe"=w426) -> (w422:T7)
                        n136 = call "3DClassificationDisplay.vi"("error in"=w424, "Parameter"=w422) -> ("error out"=w423:errorcluster)  [unwired: 9 in]
                      }
                    }
                  }
                }
                n137 = Bundle By Name(cluster=w354, "Variables.State"=State_MLPClassifier."8 - RefreshScale") -> (w367:T1)
              }
              frame "8 - RefreshScale" {
                n138 = Unbundle By Name(w433) -> ("Variables.Mode"=w434:enum32{"TRAIN", "PREDICT"}, "Variables.Representation"=w444:u32, "Variables.ScaleName"=w440:string[], "Référence.Scale 2D Pred"=w443:refnum<vi>, "Référence.Scale 3D"=w442:refnum<vi>, "Référence.Scale 2D"=w441:refnum<vi>, "Référence.GraphPred"=w439:refnum<vi>, "Référence.GraphTrain"=w438:refnum<vi>, "Référence.3D Scatter"=w437:refnum<vi>)
                n139 = case shown="0, Default" w444 {
                  tunnel: w443 -> [w447 _]
                  tunnel: w442 -> [_ w491]
                  tunnel: w441 -> [w451 _]
                  tunnel: w440 -> [w448 w488]
                  tunnel: w439 -> [w446 _]
                  tunnel: w438 -> [w450 _]
                  tunnel: w437 -> [_ w490]
                  tunnel: w436 -> [w452 w477]
                  tunnel: [w449 w476] -> w435
                  tunnel: w434 -> [w453 _]
                  frame 0, Default {
                    # "2D"
                    n140 = case shown="\"TRAIN\", Default" w453 {
                      tunnel: w452 -> [w463 w475]
                      tunnel: w451 -> [w464 _]
                      tunnel: w450 -> [w462 _]
                      tunnel: [w459 w472] -> w449
                      tunnel: w448 -> [w458 w465]
                      tunnel: w447 -> [_ w467]
                      tunnel: w446 -> [_ w466]
                      frame "TRAIN", Default {
                        n141 = property class="Clust (strict)"(reference=w464, error in=w463) -> (error out=w460:errorcluster, "Value"=w461:cluster{"X":i32, "Y":i32})  [unwired: 1 out]
                        n142 = Unbundle By Name(w461) -> ("X"=w457:i32, "Y"=w456:i32)
                        n143 = Index Array(array=w458, index #1=w457, index #2=w456) -> (element #1=w454:string, element #2=w455:string)
                        n144 = property class="XYGraph (strict)"(reference=w462, error in=w460, "XScale.NameLbl.Text"=w454, "YScale.NameLbl.Text"=w455) -> (error out=w459:errorcluster)  [unwired: 1 out]
                      }
                      frame "PREDICT" {
                        n145 = property class="Clust (strict)"(reference=w467, error in=w475) -> (error out=w473:errorcluster, "Value"=w474:cluster{"X":i32, "Y":i32})  [unwired: 1 out]
                        n146 = Unbundle By Name(w474) -> ("X"=w471:i32, "Y"=w470:i32)
                        n147 = Index Array(array=w465, index #1=w471, index #2=w470) -> (element #1=w468:string, element #2=w469:string)
                        n148 = property class="XYGraph (strict)"(reference=w466, error in=w473, "XScale.NameLbl.Text"=w468, "YScale.NameLbl.Text"=w469) -> (error out=w472:errorcluster)  [unwired: 1 out]
                      }
                    }
                  }
                  frame 1 {
                    # "3D"
                    n149 = property class="Clust (strict)"(reference=w491, error in=w477) -> (error out=w478:errorcluster, "Value"=w489:cluster{"X":i32, "Y":i32, "Z":i32})  [unwired: 1 out]
                    n150 = Unbundle By Name(w489) -> ("X"=w487:i32, "Y"=w486:i32, "Z"=w485:i32)
                    n151 = Index Array(array=w488, index #1=w487, index #2=w486, index #3=w485) -> (element #1=w480:string, element #2=w483:string, element #3=w484:string)
                    n152 = property class="3D Scatter (strict)"(reference=w490, error in=w478, "Axis:Active Axis"=enum16{"X-axis", "Y-axis", "Z-axis"}."X-axis", "Axis:Name Label Text"=w480, "Axis:Active Axis"=enum16{"X-axis", "Y-axis", "Z-axis"}."Y-axis", "Axis:Name Label Text"=w483, "Axis:Active Axis"=enum16{"X-axis", "Y-axis", "Z-axis"}."Z-axis", "Axis:Name Label Text"=w484) -> (error out=w476:errorcluster)  [unwired: 1 out]
                  }
                }
                n153 = Bundle By Name(cluster=w433, "Variables.State"=State_MLPClassifier."1 - Idle") -> (w432:T1)
              }
              frame "9 - Fit" {
                n154 = Unbundle By Name(w496) -> ("Objet.MLPClassifier"=w504:refnum<class "MLPClassifier.lvclass">, "Variables.Split.X Train"=w500:dbl[][], "Variables.Split.Y Train"=w499:dbl[][])
                n155 = property class="MLPClassifier.lvclass"(reference=w504, error in=w494, "accessors:R/W X"=w500, "accessors:R/W y"=w499) -> (reference out=w503:refnum<class "MLPClassifier.lvclass">, error out=w502:errorcluster)
                n156 = call-dynamic "fit.vi"("error in (no error)"=w502, "MultiLayerPerceptron.lvclass 2"=w503) -> ("error out"=w498:errorcluster, "MultiLayerPerceptron.lvclass"=w501:refnum<class "MLPClassifier.lvclass">)  [unwired: 8 in]
                n157 = Bundle By Name(cluster=w496, "Variables.State"=State_MLPClassifier."10 - Predict", "Objet.MLPClassifier"=w501, "Variables.Train ?"=TRUE) -> (w493:T1)
              }
              frame "10 - Predict" {
                n158 = Unbundle By Name(w510) -> ("Variables.Mode"=w513:enum32{"TRAIN", "PREDICT"}, "Objet.MLPClassifier"=w509:refnum<class "MLPClassifier.lvclass">, "Variables.Split.X Test"=w507:dbl[][], "Variables.Split.Y Test"=w506:dbl[][], "Variables.X"=w505:dbl[][])
                n159 = case shown="\"TRAIN\", Default" w513 {
                  tunnel: w507 -> [w517 _]
                  tunnel: w508 -> [w515 w540]
                  tunnel: [w527 w537] -> w512
                  tunnel: w509 -> [w521 w541]
                  tunnel: [w535 w546] -> w511
                  tunnel: w510 -> [w524 w544]
                  tunnel: w506 -> [w516 _]
                  tunnel: w505 -> [_ w536]
                  frame "TRAIN", Default {
                    n160 = property class="MLPClassifier.lvclass"(reference=w521, error in=w515, "accessors:R/W X"=w517, "accessors:R/W y"=w516) -> (reference out=w520:refnum<class "MLPClassifier.lvclass">, error out=w523:errorcluster)
                    n161 = call-dynamic "predict.vi"("error in (no error)"=w523, "MultiLayerPerceptron.lvclass 2"=w520) -> ("error out"=w518:errorcluster, "C"=w522:dbl[][], "MultiLayerPerceptron.lvclass"=w519:refnum<class "MLPClassifier.lvclass">)  [unwired: 7 in]
                    n162 = call-dynamic "score.vi"("error in (no error)"=w518, "MultiLayerPerceptron.lvclass 2"=w519) -> ("error out"=w527:errorcluster, "score"=→"Score":dbl, "MultiLayerPerceptron.lvclass"=w529:refnum<class "MLPClassifier.lvclass">)  [unwired: 7 in]
                    n163 = Index Array(array=w516, index (col)=0 ("disabled index (col)")) -> (element=w530:dbl[])  [unwired: 1 in]
                    n164 = Index Array(array=w522, index (col)=0 ("disabled index (col)")) -> (element=w532:dbl[])  [unwired: 1 in]
                    n165 = call "Rating.vi"("Class Predict"=w532, "Class Real"=w530) -> ("Bad"=→"Bad":i32, "Good"=→"Good":i32)  [unwired: 8 in]
                    n166 = Bundle By Name(cluster=w524, "Variables.FitPredict"=w522, "Objet.MLPClassifier"=w529, "Variables.State"=State_MLPClassifier."7 - DisplayDataTrain") -> (w535:T1)
                  }
                  frame "PREDICT" {
                    n167 = property class="MLPClassifier.lvclass"(reference=w541, error in=w540, "accessors:R/W X"=w536) -> (reference out=w542:refnum<class "MLPClassifier.lvclass">, error out=w543:errorcluster)
                    n168 = call-dynamic "predict.vi"("error in (no error)"=w543, "MultiLayerPerceptron.lvclass 2"=w542) -> ("error out"=w537:errorcluster, "C"=w538:dbl[][], "MultiLayerPerceptron.lvclass"=w539:refnum<class "MLPClassifier.lvclass">)  [unwired: 7 in]
                    "Prediction" <- w538
                    n169 = Bundle By Name(cluster=w544, "Variables.Predict"=w538, "Objet.MLPClassifier"=w539, "Variables.State"=State_MLPClassifier."14 - DisplayDataPredict") -> (w546:T1)
                  }
                }
              }
              frame "11 - SetParameters" {
                n170 = Unbundle By Name(w552) -> ("Objet.MLPClassifier"=w558:refnum<class "MLPClassifier.lvclass">)
                n171 = call "SettingParameters.vi"("error in"=w551) -> ("error out"=w554:errorcluster, "Parameters"=w553:T10)  [unwired: 9 in]
                n172 = property class="MLPClassifier.lvclass"(reference=w558, error in=w554, "accessors:R/W params"=w553) -> (reference out=w555:refnum<class "MLPClassifier.lvclass">, error out=w557:errorcluster)
                n173 = call-dynamic "set_params.vi"("error in (no error)"=w557, "MLPClassifier.lvclass 2"=w555) -> ("error out"=w550:errorcluster, "MLPClassifier.lvclass"=w556:refnum<class "MLPClassifier.lvclass">)  [unwired: 8 in]
                n174 = Bundle By Name(cluster=w552, "Variables.State"=State_MLPClassifier."1 - Idle", "Objet.MLPClassifier"=w556) -> (w548:T1)
              }
              frame "12 - SaveModel" {
                n175 = Unbundle By Name(w559) -> ("Variables.Model Name"=w562:string, "Objet.MLPClassifier"=w567:refnum<class "MLPClassifier.lvclass">)
                n176 = Get Date/Time In Seconds() -> (seconds since 1Jan1904=w565:timestamp)
                n177 = Format Date/Time String(time format string (%c)="%Y%m%d_", seconds (now)=w565) -> (date/time string=w563:string)  [unwired: 1 in]
                n178 = Concatenate Strings(w563, " " ("string"), w562) -> (w560:string)
                n179 = call "File Dialog2"("default name"=w560, "error in"=w571) -> ("selected path"=w572:path, "cancelled"=w573:bool, "error out"=w574:errorcluster)  [unwired: 10 in, 1 out]
                n180 = case shown="False" w573 {
                  tunnel: [w588 w590] -> w570
                  tunnel: w574 -> [w577 w591]
                  tunnel: w572 -> [w587 _]
                  tunnel: w567 -> [w585 w589]
                  tunnel: [w586 w589] -> w568
                  frame False {
                    n181 = Path To String(path=w587) -> (string=w582:string)
                    n182 = Search and Replace String(replace all?=TRUE ("replace all? (F)"), input string=w582, search string="\\", replace string="/" ("replace string (\"\")"), error in=w577) -> (result string=w578:string, error out=w576:errorcluster)  [unwired: 3 in, 2 out]
                    n183 = property class="MLPClassifier.lvclass"(reference=w585, error in=w576, "accessors:save_path"=w578) -> (reference out=w584:refnum<class "MLPClassifier.lvclass">, error out=w583:errorcluster)
                    n184 = call-dynamic "save.vi"("error in (no error)"=w583, "Model.lvclass"=w584) -> ("error out"=w588:errorcluster, "Model.lvclass 2"=w586:refnum<class "MLPClassifier.lvclass">)  [unwired: 7 in, 1 out]
                  }
                  frame True {
                    n185 = call <vilib>:"Clear Errors.vi"("error in (no error)"=w591) -> ("error out"=w590:errorcluster)  [unwired: 5 in, 1 out]
                  }
                }
                n186 = Bundle By Name(cluster=w559, "Variables.State"=State_MLPClassifier."1 - Idle", "Objet.MLPClassifier"=w568) -> (w566:T1)
              }
              frame "13 - LoadModel" {
                n187 = Unbundle By Name(w593) -> ("Variables.Model Name"=w594:string, "Objet.MLPClassifier"=w598:refnum<class "MLPClassifier.lvclass">)
                n188 = Concatenate Strings("Load " ("string"), w594) -> (w595:string)
                n189 = call "File Dialog"("prompt"=w595, "error in"=w602, "pattern (all files)"="*.gz") -> ("selected path"=w599:path, "cancelled"=w600:bool, "error out"=w601:errorcluster)  [unwired: 9 in, 1 out]
                n190 = case shown="False" w600 {
                  tunnel: [w620 w625] -> w603
                  tunnel: w601 -> [w607 w626]
                  tunnel: w599 -> [w608 _]
                  tunnel: w598 -> [w615 w623]
                  tunnel: w593 -> [w619 w624]
                  tunnel: [w618 w622] -> w592
                  frame False {
                    n191 = Path To String(path=w608) -> (string=w612:string)
                    n192 = Search and Replace String(replace all?=TRUE ("replace all? (F)"), input string=w612, search string="\\", replace string="/" ("replace string (\"\")"), error in=w607) -> (result string=w609:string, error out=w606:errorcluster)  [unwired: 3 in, 2 out]
                    n193 = property class="MLPClassifier.lvclass"(reference=w615, error in=w606, "accessors:load_path"=w609) -> (reference out=w614:refnum<class "MLPClassifier.lvclass">, error out=w613:errorcluster)
                    n194 = call-dynamic "load.vi"("error in (no error)"=w613, "Model.lvclass"=w614) -> ("error out"=w620:errorcluster, "Model.lvclass 2"=w617:refnum<class "MLPClassifier.lvclass">)  [unwired: 7 in, 1 out]
                    n195 = Bundle By Name(cluster=w619, "Variables.State"=State_MLPClassifier."1 - Idle", "Objet.MLPClassifier"=w617) -> (w618:T1)
                  }
                  frame True {
                    n196 = call <vilib>:"Clear Errors.vi"("error in (no error)"=w626) -> ("error out"=w625:errorcluster)  [unwired: 5 in, 1 out]
                    n197 = Bundle By Name(cluster=w624, "Variables.State"=State_MLPClassifier."1 - Idle", "Objet.MLPClassifier"=w623) -> (w622:T1)
                  }
                }
              }
              frame "14 - DisplayDataPredict" {
                n198 = Unbundle By Name(w639) -> ("Variables.X"=w632:dbl[][], "Variables.Predict"=w633:dbl[][], "Référence.GraphPred"=w634:refnum<vi>, "Référence.Scale 2D Pred"=w635:refnum<vi>)
                n199 = property class="Clust (strict)"(reference=w635, error in=w627) -> (error out=w631:errorcluster, "Value"=w636:cluster{"X":i32, "Y":i32})  [unwired: 1 out]
                n200 = Bundle By Name(cluster=T8 {"Plot"=refnum, "Data"={"X"=[], "Predict"=[]}, "Indexe"={"X"=0, "Y"=1}, "Point Property"={"Style"=enum."Full circle", "Label Color"=[8978528, 4367871, 1985280]}} ("Parameters"), "Data.X"=w632, "Data.Predict"=w633, "Plot"=w634, "Indexe"=w636) -> (w629:T8)
                n201 = Bundle By Name(cluster=w639, "Variables.State"=State_MLPClassifier."8 - RefreshScale") -> (w638:T1)
                n202 = call "2DPredictedClassification.vi"("error in"=w631, "Parameters"=w629) -> ("error out"=w628:errorcluster)  [unwired: 9 in]
              }
              frame "Error" {
                n203 = Unbundle By Name(w643) -> ("code"=w641:i32)
                n204 = case shown="1672" w641 {
                  tunnel: [w652 w661] -> w646
                  tunnel: w643 -> [w651 w657]
                  tunnel: w644 -> [w650 w656]
                  tunnel: [w648 w659] -> w642
                  frame Default {
                    n205 = call <vilib>:"Simple Error Handler.vi"("error in (no error)"=w651) -> ("error out"=w647:errorcluster)  [unwired: 4 in, 4 out]
                    n206 = Bundle By Name(cluster=w650, "Variables.State"=State_MLPClassifier."Exit") -> (w648:T1)
                    n207 = call <vilib>:"Clear Errors.vi"("error in (no error)"=w647) -> ("error out"=w652:errorcluster)  [unwired: 5 in, 1 out]
                  }
                  frame 1672 {
                    n208 = Unbundle By Name(w656) -> ("Objet.MLPClassifier"=w658:refnum<class "MLPClassifier.lvclass">)
                    n209 = call "debug.vim"("error in (no error)"=w657, "Model.lvclass"=w658) -> ("error out"=w655:errorcluster, "standard error"=w653:string, "reference out"=w654:refnum<class "MLPClassifier.lvclass">)  [unwired: 7 in]
                    n210 = Bundle By Name(cluster=w656, "Variables.State"=State_MLPClassifier."1 - Idle", "Objet.MLPClassifier"=w654) -> (w659:T1)
                    n211 = One Button Dialog(message=w653) -> ()  [unwired: 1 in, 1 out]
                    n212 = call <vilib>:"Clear Errors.vi"("error in (no error)"=w655) -> ("error out"=w661:errorcluster)  [unwired: 5 in, 1 out]
                  }
                }
              }
              frame "Exit" {
                n213 = Unbundle By Name(w662) -> ("Objet.MLPClassifier"=w665:refnum<class "MLPClassifier.lvclass">)
                n214 = call-dynamic "closeSession.vi"("error in"=w664, "Python en entrée"=w665) -> ("error out"=w663:errorcluster)  [unwired: 8 in, 1 out]
              }
            }
            n215 = case shown="No Error" w21 {
              selector: w21 -> [w668 w671]
              tunnel: [w668 w671] -> w20
              tunnel: w17 -> [w667 w672]
              tunnel: [w667 w670] -> w16
              frame No Error {
              }
              frame Error {
                n216 = Bundle By Name(cluster=w672, "Variables.State"=State_MLPClassifier."Error" ("State")) -> (w670:T1)
              }
            }
          }
        }
      }
    }
    frame Error {
    }
  }
  "error out" <- w1
